vi "Initialize AO Channels.vi"(8 "error in (no error)":errorcluster, 11 "Instrument.DAQ":refnum<class "Instrument.DAQ.lvclass">) -> (0 "error out":errorcluster, 3 "Instrument.DAQ out":refnum<class "Instrument.DAQ.lvclass">)   [LabVIEW 2019, in "Instrument.Lockin.lvlib" / "Instrument.DAQ.lvclass"]
uses:
  Instrument.DAQ.lvclass
  Instrument.DAQ.lvclass/Instrument.DAQ.ctl
panel:
  # "1"
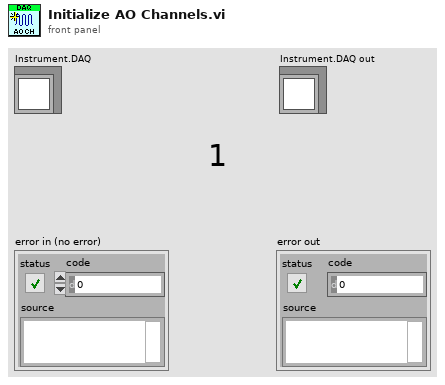
[diagram p1: front panel]
types:
  T1 = typedef "Instrument.Lockin.lvlib/Instrument.DAQ.lvclass/AO.Channel--Cluster--Array.ctl" = T2[]
  T2 = typedef "Instrument.Lockin.lvlib/Instrument.DAQ.lvclass/AO.Channel--Cluster.ctl" = cluster{"Enable?":bool, "Channel":i32, "Amplitude":dbl, "Offset":dbl, "Frequency":dbl, "Phase":dbl, "Function":T3, "Sweeping?":bool, "Limit AC":bool, "Limit DC?":bool, "Duty Cycle":bool}
  T3 = typedef "Instrument.Lockin.lvlib/Instrument.DAQ.lvclass/AO.Channel.Function--Enum.ctl" = enum16{"sine", "square", "triangle", "saw"}
  T4 = typedef "Instrument.Lockin.lvlib/Instrument.DAQ.lvclass/DAQ.Config.AO--Cluster--Array.ctl" = cluster{"Channels":tag, "Range":T5, "terminal configuration":T6, "Type":T7}[]
  T5 = typedef "Instrument.Lockin.lvlib/Instrument.DAQ.lvclass/DAQ.Config.AO.Range--enum.ctl" = enum16{"±0.1", "±1.0", "±3.5", "±10.0", ""}
  T6 = typedef "Instrument.Lockin.lvlib/Instrument.DAQ.lvclass/DAQ.TerminalConfiguration--ring.ctl" = i32
  T7 = typedef "Instrument.Lockin.lvlib/Instrument.DAQ.lvclass/DAQ.Type--enum.ctl" = enum16{"None", "USB-4431", "PXI-446x"}
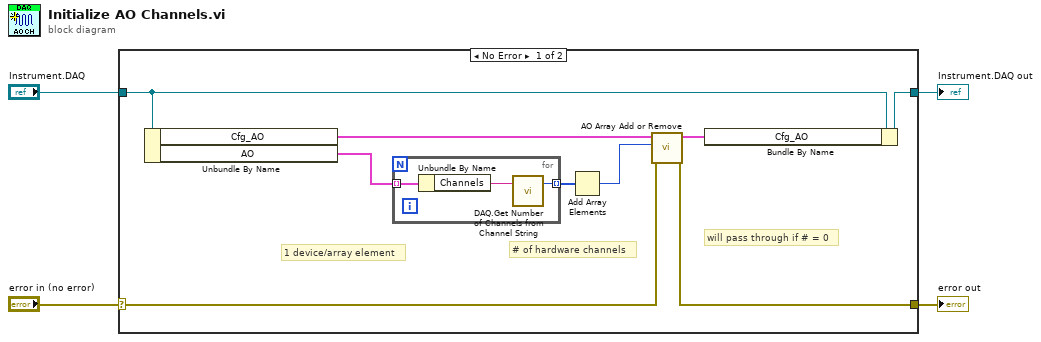
[diagram p0: block diagram]
diagram:
  n1 = case shown="No Error" "error in (no error)" {
    selector: "error in (no error)" -> [w10 w18]
    tunnel: "Instrument.DAQ" -> [w12 w17]
    tunnel: [w11 w17] -> w3
    tunnel: [w9 w18] -> w1
    frame No Error {
      # "will pass through if # = 0"
      # "1 device/array element"
      # "# of hardware channels"
      n2 = Unbundle By Name(w12) -> ("Cfg_AO"=w8:T1, "AO"=w7:T4)
      n3 = for {
        tunnel: w7 -> [w16] mode=indexing
        tunnel: [w15] -> w13 mode=indexing
        n4 = Unbundle By Name(w16) -> ("Channels"=w14:tag)
        n5 = call "DAQ.Get Number of Channels from Channel String.vi"("Channels String"=w14) -> ("# channels"=w15:i32)  [unwired: 2 in]
      }
      n6 = Add Array Elements(numeric array=w13) -> (sum=w5:i32)
      n7 = call "AO Array Add or Remove.vi"("error in (no error)"=w10, "Size"=w5, "AO Channels in"=w8) -> ("error out"=w9:errorcluster, "AO Channels out"=w6:T1)  [unwired: 7 in]
      n8 = Bundle By Name(cluster=w12, "Cfg_AO"=w6) -> (w11:refnum<class "Instrument.DAQ.lvclass">)
    }
    frame Error {
    }
  }
  "Instrument.DAQ out" <- w3
  "error out" <- w1
